vi "Handle Notification.vi"(8 "error in (no error)":errorcluster, 9 "Payload":string, 10 "Notification Type":string, 11 "Performanced XNET CAN Signal Logger in":refnum<class "Performanced XNET CAN Signal Logger.lvclass">) -> (0 "error out":errorcluster, 3 "Performanced XNET CAN Signal Logger out":refnum<class "Performanced XNET CAN Signal Logger.lvclass">)   [LabVIEW 2021, in "Performanced XNET CAN Signal Logger.lvlib" / "Performanced XNET CAN Signal Logger.lvclass"]
uses:
  Performanced XNET CAN Signal Logger.lvclass
  Typedef/Def-Executor Command.ctl
  XNET-CAN-Signal-Logger.lvlib
  <vilib>/FlexLogger/SDK/PluginSDK.lvlibp/PEFClasses/SDK/Plugin/Plugin.lvclass
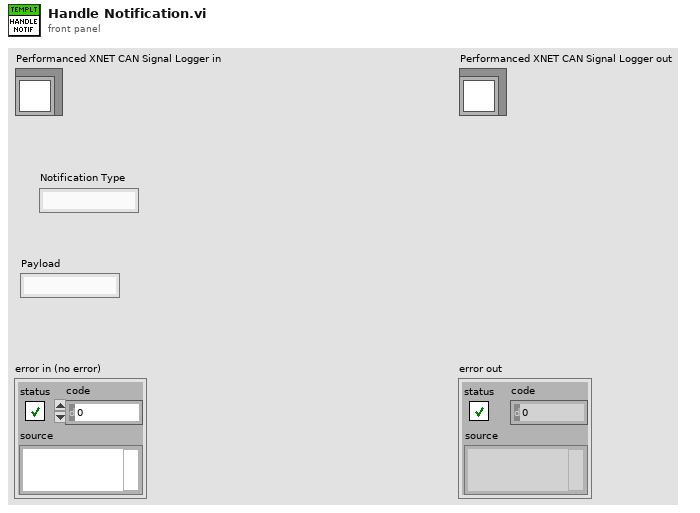
[diagram p1: front panel]
types:
  T1 = typedef "XNET-CAN-Signal-Logger.lvlib/Def-Executor Command.ctl" = cluster{"Command":string, "Data":variant}
  T2 = typedef "XNET-CAN-Signal-Logger.lvlib/Def-LogSpec.ctl" = cluster{"Log file folder":path, "Log file name":string, "Segment Files":bool, "Segment File Size":i64}
  T3 = typedef "XNET-CAN-Signal-Logger.lvlib/Def-CAN Port Configuration.ctl" = cluster{"CAN Interface":refnum<k21>, "XNET Cluster":refnum<k21>, "#Signals":i32, "Sample Rate (Hz)":dbl}
  T4 = cluster{"LogSpec out":T2, "CAN Configurations out":T3[]}
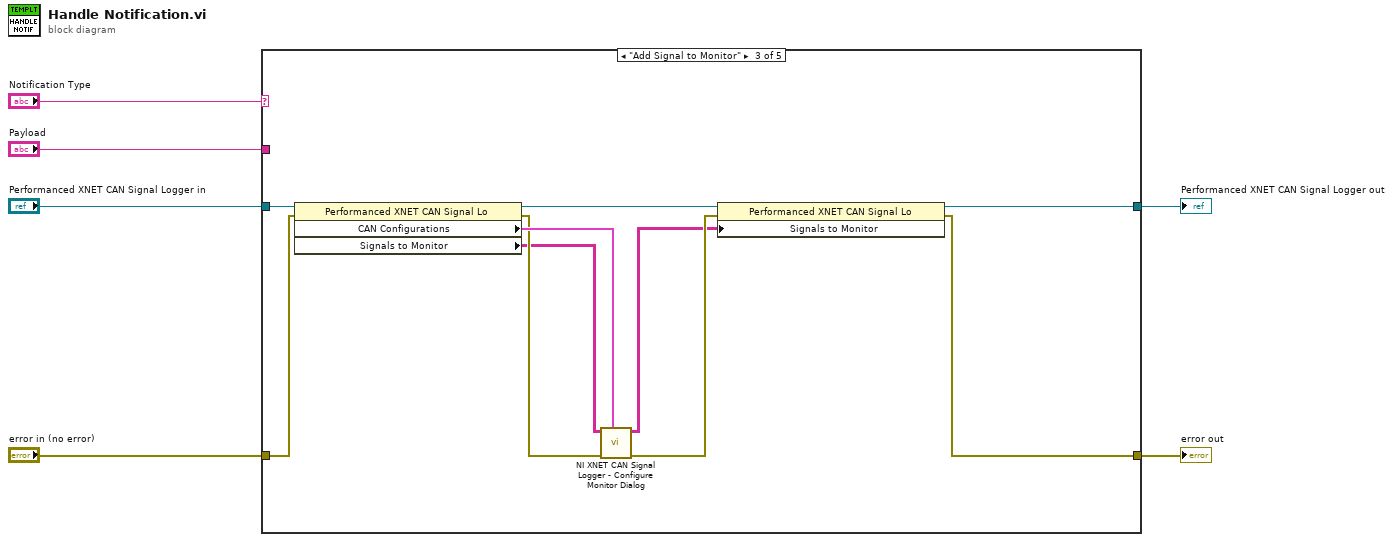
[diagram p0: block diagram]
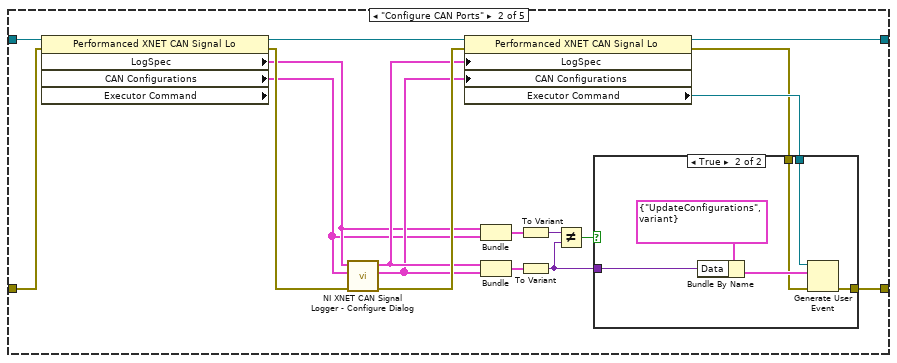
[diagram p3: hidden frame]
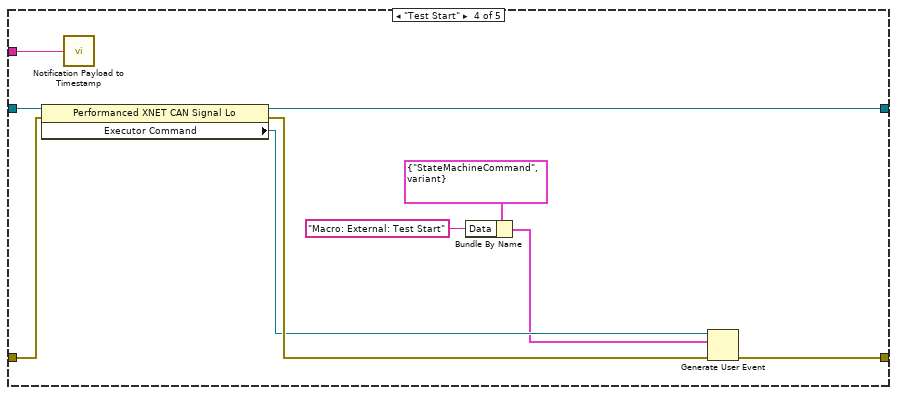
[diagram p5: hidden frame]
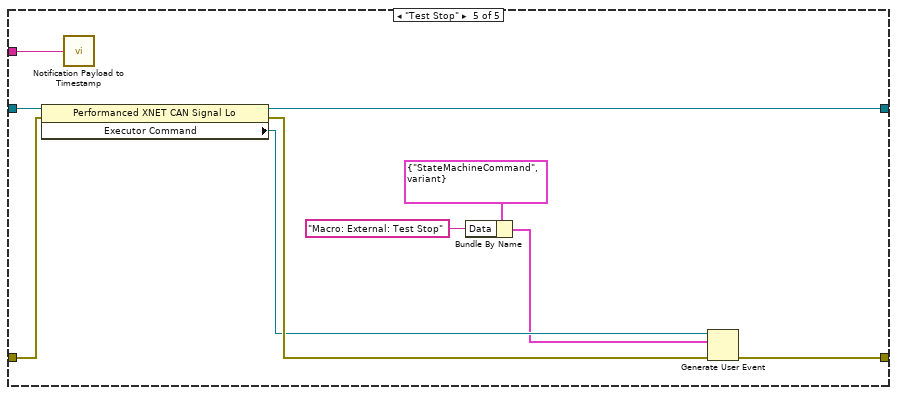
[diagram p6: hidden frame]
diagram:
  n1 = case shown="\"Add Signal to Monitor\"" "Notification Type" {
    tunnel: [w8 w9 w36 w49 w59] -> w1
    tunnel: "error in (no error)" -> [w8 w23 w39 w51 w61]
    tunnel: "Payload" -> [_ _ _ w44 w54]
    tunnel: [w7 w24 w41 w52 w62] -> w3
    tunnel: "Performanced XNET CAN Signal Logger in" -> [w7 w26 w43 w53 w63]
    frame Default {
    }
    frame "Configure CAN Ports" {
      n2 = property class="Performanced XNET CAN Signal Lo" props=["LogSpec", "CAN Configurations", "Executor Command"](reference=w26, error in=w23) -> (reference out=w25:refnum<class "Performanced XNET CAN Signal Logger.lvclass">, error out=w22:errorcluster, "LogSpec"=w15:T2, "CAN Configurations"=w14:T3[])  [unwired: 1 out]
      n3 = call "NI XNET CAN Signal Logger - Configure Dialog.vi"("error in (no error)"=w22, "CAN Configurations in"=w14, "LogSpec in"=w15) -> ("error out"=w21:errorcluster, "CAN Configurations out"=w18:T3[], "LogSpec out"=w19:T2)  [unwired: 6 in]
      n4 = property class="Performanced XNET CAN Signal Lo"(reference=w25, error in=w21, "LogSpec"=w19, "CAN Configurations"=w18) -> (reference out=w24:refnum<class "Performanced XNET CAN Signal Logger.lvclass">, error out=w10:errorcluster, "Executor Command"=w20:refnum<user-event>)
      n5 = Bundle("LogSpec"=w15, "CAN Configurations"=w14) -> (w17:cluster{"LogSpec":T2, "CAN Configurations":T3[]})  [unwired: 1 in]
      n6 = Bundle("LogSpec out"=w19, "CAN Configurations out"=w18) -> (w16:T4)  [unwired: 1 in]
      n7 = To Variant(anything=w17) -> (Variant=w13:variant)
      n8 = To Variant(anything=w16) -> (Variant=w12:variant)
      n9 = Not Equal?(x=w13, y=w12) -> (x != y?=w11:bool)
      n10 = case shown="True" w11 {
        tunnel: w20 -> [_ w31]
        tunnel: w12 -> [_ w30]
        tunnel: w10 -> [w27 w29]
        tunnel: [w27 w28] -> w9
        frame False {
        }
        frame True {
          n11 = Bundle By Name(cluster=T1 {"Command"="UpdateConfigurations", "Data"=variant} ("event data"), "Data"=w30) -> (w32:T1)
          n12 = Generate User Event(user event=w31, event data cluster=w32, error in=w29) -> (error out=w28:errorcluster)  [unwired: 1 in, 1 out]
        }
      }
    }
    frame "Add Signal to Monitor" {
      n13 = property class="Performanced XNET CAN Signal Lo"(reference=w43, error in=w39) -> (reference out=w42:refnum<class "Performanced XNET CAN Signal Logger.lvclass">, error out=w38:errorcluster, "CAN Configurations"=w40:T3[], "Signals to Monitor"=w35:string[][])
      n14 = call "NI XNET CAN Signal Logger - Configure Monitor Dialog.vi"("CAN Configurations"=w40, "error in (no error)"=w38, "Signal to Monitor in"=w35) -> ("error out"=w37:errorcluster, "Signal to Monitor out"=w34:string[][])  [unwired: 7 in]
      n15 = property class="Performanced XNET CAN Signal Lo"(reference=w42, error in=w37, "Signals to Monitor"=w34) -> (reference out=w41:refnum<class "Performanced XNET CAN Signal Logger.lvclass">, error out=w36:errorcluster)
    }
    frame "Test Start" {
      n16 = property class="Performanced XNET CAN Signal Lo"(reference=w53, error in=w51) -> (reference out=w52:refnum<class "Performanced XNET CAN Signal Logger.lvclass">, error out=w50:errorcluster, "Executor Command"=w48:refnum<user-event>)
      n17 = call <vilib>:"Notification Payload to Timestamp.vi"("Payload"=w44) -> ()  [unwired: 1 out]
      n18 = Bundle By Name(cluster=T1 {"Command"="StateMachineCommand", "Data"=variant} ("event data"), "Data"="Macro: External: Test Start") -> (w46:T1)
      n19 = Generate User Event(user event=w48, event data cluster=w46, error in=w50) -> (error out=w49:errorcluster)  [unwired: 1 in, 1 out]
    }
    frame "Test Stop" {
      n20 = property class="Performanced XNET CAN Signal Lo"(reference=w63, error in=w61) -> (reference out=w62:refnum<class "Performanced XNET CAN Signal Logger.lvclass">, error out=w60:errorcluster, "Executor Command"=w58:refnum<user-event>)
      n21 = call <vilib>:"Notification Payload to Timestamp.vi"("Payload"=w54) -> ()  [unwired: 1 out]
      n22 = Bundle By Name(cluster=T1 {"Command"="StateMachineCommand", "Data"=variant} ("event data"), "Data"="Macro: External: Test Stop") -> (w56:T1)
      n23 = Generate User Event(user event=w58, event data cluster=w56, error in=w60) -> (error out=w59:errorcluster)  [unwired: 1 in, 1 out]
    }
  }
  "error out" <- w1
  "Performanced XNET CAN Signal Logger out" <- w3
